vi "Actor Stopped.vi"(8 "error in (no error)":errorcluster, 10 "Actor's Self Q":refnum<class "Message Enqueuer.lvclass">, 11 "Actor Monitor New in":refnum<class "Actor Monitor.lvclass">) -> (0 "error out":errorcluster, 3 "Actor Monitor New out":refnum<class "Actor Monitor.lvclass">)   [LabVIEW 2023, in "Monitored Actor.lvlib" / "Actor Monitor.lvclass"]
doc: "Removes the Actor from the monitored data object\n\nCopyright: MGI 2016\nAuthor: Derek Trepanier"
uses:
  Actor Monitor.lvclass
  C:/Users/Public/Documents/Development/builds/Engine/Actor Framework.lvlibp/1abvi3w/vi.lib/ActorFramework/Actor/Actor.lvclass
  builds/Engine/Actor Framework.lvlibp/1abvi3w/vi.lib/ActorFramework/Message Enqueuer/Message Enqueuer.lvclass
  Actor Monitor.lvclass/Actor Monitor.ctl
  Monitor Data/Monitor Data.lvclass
  builds/Engine/Actor Framework.lvlibp/1abvi3w/vi.lib/ActorFramework/Stop Msg/Stop Msg.lvclass
  builds/Engine/Actor Framework.lvlibp/1abvi3w/vi.lib/ActorFramework/Actor/Actor.lvclass
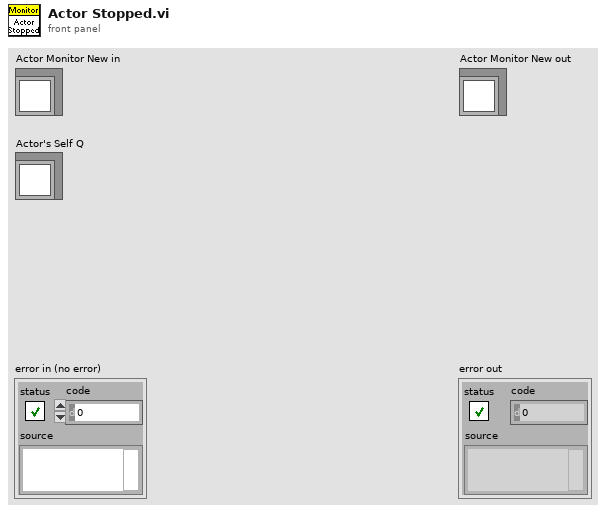
[diagram p1: front panel]
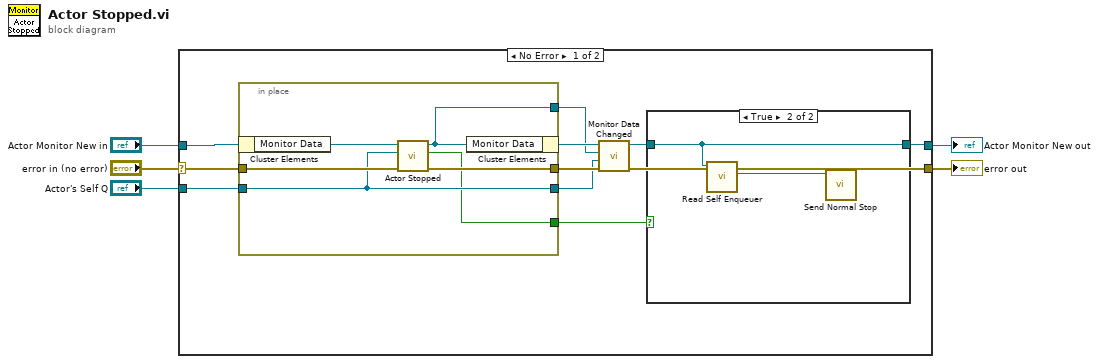
[diagram p0: block diagram]
diagram:
  n1 = case shown="No Error" "error in (no error)" {
    selector: "error in (no error)" -> [w14 w27]
    tunnel: [w12 w27] -> w4
    tunnel: [w6 w26] -> w2
    tunnel: "Actor Monitor New in" -> [w16 w26]
    tunnel: "Actor's Self Q" -> [w13 _]
    frame No Error {
      n2 = in-place {
        in-place-border: [w24] -> w15
        in-place-border: w14 -> [w23]
        in-place-border: w13 -> [w22]
        in-place-border: [w21] -> w10
        in-place-border: [w22] -> w9
        in-place-border: [w20] -> w7
        n3 = in-place-cluster #1(w16) -> ("Monitor Data"=w25:refnum<class "Monitor Data.lvclass">)
        n4 = call "Actor Stopped.vi"("error in (no error)"=w23, "Actor's Self Q"=w22, "Monitor Data in"=w25) -> ("error out"=w24:errorcluster, "Empty?"=w20:bool, "Monitor Data out"=w21:refnum<class "Monitor Data.lvclass">)  [unwired: 6 in]
        n5 = in-place-cluster #1("Monitor Data"=w21) -> (w11:refnum<class "Actor Monitor.lvclass">)
      }
      n6 = call-dynamic "Monitor Data Changed.vi"("error in (no error)"=w15, "Changed Actor's Q"=w9, "Monitor Data"=w10, "Actor Monitor New in"=w11) -> ("error out"=w12:errorcluster, "Actor Monitor New out"=w8:refnum<class "Actor Monitor.lvclass">)  [unwired: 6 in]
      n7 = case shown="True" w7 {
        tunnel: w8 -> [w17 w19]
        tunnel: [w17 w19] -> w6
        frame False {
        }
        frame True {
          n8 = call "Read Self Enqueuer.vi"("Actor"=w19) -> ("Self Enqueuer"=w18:refnum<class "Message Enqueuer.lvclass">)  [unwired: 10 in]
          n9 = call "Send Normal Stop.vi"("Message Enqueuer"=w18) -> ()  [unwired: 10 in, 1 out]
        }
      }
    }
    frame Error {
    }
  }
  "error out" <- w4
  "Actor Monitor New out" <- w2
